vi "Wiimote Get Core Buttons, Acceleration, IR Sensor and Extension Controller.vi"(8 "error in":errorcluster, 11 "hWiimoteHandle in":u32 format="%08x") -> (0 "error out":errorcluster, 2 "Data out":T6, 3 "hWiimoteHandle out":u32 format="%08x")   [LabVIEW 2012, in "Wiimote.lvlib"]
uses:
  Wiimote.lvlib
  Wiimote Buttons.ctl
  Wiimote Acceleration.ctl
  Wiimote IR Sensor.ctl
  Wiimote Point.ctl
  Nunchuk Buttons.ctl
  Wiimote Reporting Mode.ctl
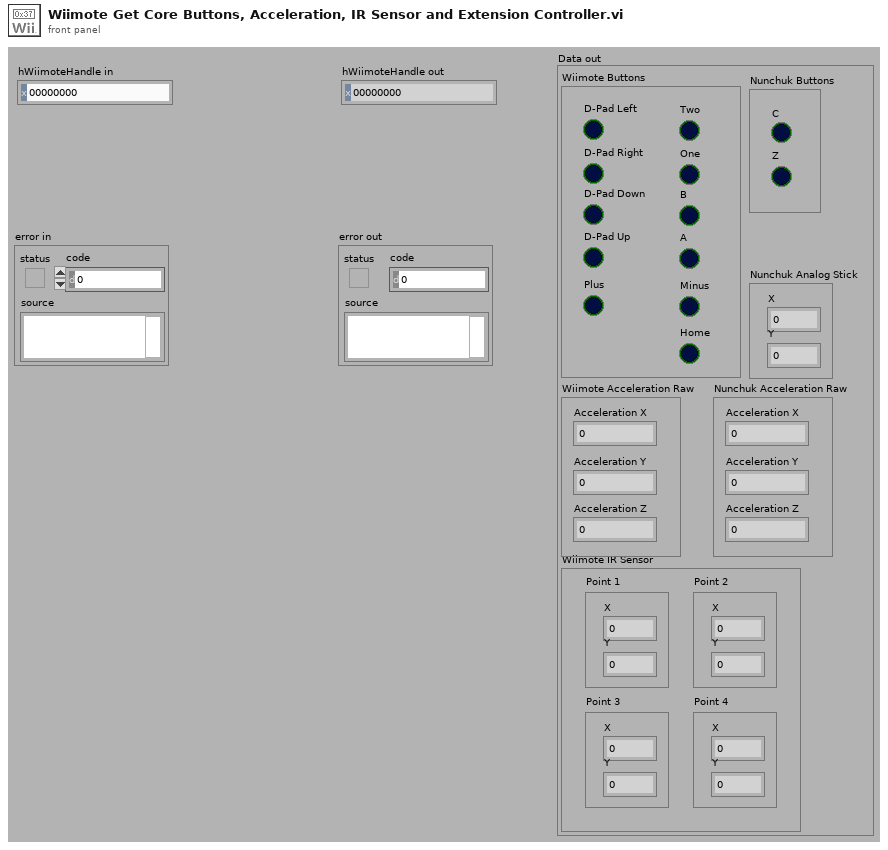
[diagram p1: front panel]
types:
  T1 = typedef "Wiimote.lvlib/Wiimote Buttons.ctl" = cluster{"D-Pad Left":bool, "D-Pad Right":bool, "D-Pad Down":bool, "D-Pad Up":bool, "Plus":bool, "Two":bool, "One":bool, "B":bool, "A":bool, "Minus":bool, "Home":bool}
  T2 = typedef "Wiimote.lvlib/Wiimote Acceleration.ctl" = cluster{"Acceleration X":dbl, "Acceleration Y":dbl, "Acceleration Z":dbl}
  T3 = typedef "Wiimote.lvlib/Wiimote IR Sensor.ctl" = cluster{"Point 1":T4, "Point 2":T4, "Point 3":T4, "Point 4":T4}
  T4 = typedef "Wiimote.lvlib/Wiimote Point.ctl" = cluster{"X":u16, "Y":u16}
  T5 = typedef "Wiimote.lvlib/Nunchuk Buttons.ctl" = cluster{"C":bool, "Z":bool}
  T6 = cluster{"Wiimote Buttons":T1, "Wiimote Acceleration Raw":T2, "Wiimote IR Sensor":T3, "Nunchuk Analog Stick":T4, "Nunchuk Acceleration Raw":T2, "Nunchuk Buttons":T5}
  T7 = typedef "Wiimote.lvlib/Wiimote Reporting Mode.ctl" = u8
  T8 = cluster{"Wiimote Buttons out":T1, "Wiimote Acceleration Raw out":T2, "Wiimote IR Sensor out":T3, "Nunchuk Analog Stick out":T4, "Nunchuk Acceleration Raw out":T2, "Nunchuk Buttons out":T5}
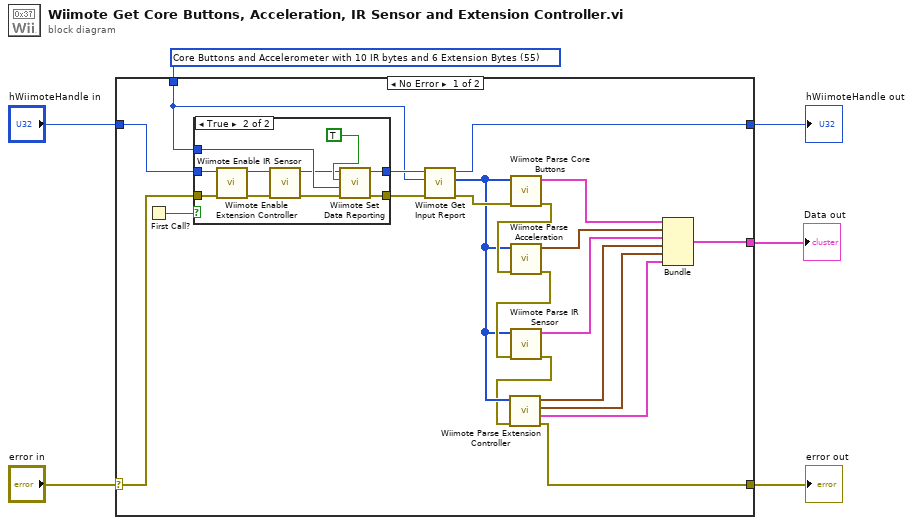
[diagram p0: block diagram]
diagram:
  w2 = T7 55 items=["Core Buttons"=48, "Core Buttons and Accelerometer"=49, "Core Buttons with 8 Extension bytes"=50, "Core Buttons and Accelerometer with 12 IR bytes"=51, "Core Buttons with 19 Extension bytes"=52, "Core Buttons and Accelerometer with 16 Extension Bytes"=53, "Core Buttons with 10 IR bytes and 9 Extension Bytes"=54, "Core Buttons and Accelerometer with 10 IR bytes and 6 Extension Bytes"=55] ("Reporting Mode")
  n1 = case shown="No Error" "error in" {
    selector: "error in" -> [w19 w40]
    tunnel: [w14 w40] -> w5
    tunnel: "hWiimoteHandle in" -> [w20 w39]
    tunnel: [w25 w39] -> w3
    tunnel: w2 -> [w21 _]
    tunnel: [w7 _] -> w1
    frame No Error {
      n2 = First Call?() -> (First Call?: T/F=w18:bool)
      n3 = case shown="True" w18 {
        tunnel: [w28 w33] -> w23
        tunnel: [w27 w29] -> w22
        tunnel: w21 -> [_ w38]
        tunnel: w20 -> [w28 w36]
        tunnel: w19 -> [w27 w32]
        frame False {
        }
        frame True {
          n4 = call "Wiimote Enable Extension Controller.vi"("error in"=w32, "hWiimoteHandle in"=w36) -> ("error out"=w31:errorcluster, "hWiimoteHandle out"=w35:u32)  [unwired: 8 in]
          n5 = call "Wiimote Enable IR Sensor.vi"("error in"=w31, "hWiimoteHandle in"=w35) -> ("error out"=w30:errorcluster, "hWiimoteHandle out"=w34:u32)  [unwired: 8 in]
          n6 = call "Wiimote Set Data Reporting.vi"("error in"=w30, "Reporting Mode"=w38, "Continuous"=TRUE, "hWiimoteHandle in"=w34) -> ("error out"=w29:errorcluster, "hWiimoteHandle out"=w33:u32)  [unwired: 6 in]
        }
      }
      n7 = call "Wiimote Get Input Report.vi"("error in"=w22, "bInputReport"=w21, "hWiimoteHandle in"=w23) -> ("error out"=w26:errorcluster, "pReportBuffer out"=w16:u8[], "hWiimoteHandle out"=w25:u32)  [unwired: 6 in]
      n8 = call "Wiimote Parse Core Buttons.vi"("error in"=w26, "pReportBuffer in"=w16) -> ("error out"=w24:errorcluster, "Wiimote Buttons out"=w13:T1)  [unwired: 8 in]
      n9 = call "Wiimote Parse Acceleration.vi"("error in"=w24, "pReportBuffer in"=w16) -> ("error out"=w17:errorcluster, "Wiimote Acceleration Raw out"=w12:T2)  [unwired: 8 in]
      n10 = call "Wiimote Parse IR Sensor.vi"("error in"=w17, "pReportBuffer in"=w16) -> ("error out"=w15:errorcluster, "Wiimote IR Sensor out"=w11:T3)  [unwired: 8 in]
      n11 = call "Wiimote Parse Extension Controller.vi"("error in"=w15, "pReportBuffer in"=w16) -> ("error out"=w14:errorcluster, "Nunchuk Buttons out"=w8:T5, "Nunchuk Acceleration Raw out"=w9:T2, "Nunchuk Analog Stick out"=w10:T4)  [unwired: 6 in]
      n12 = Bundle("Wiimote Buttons out"=w13, "Wiimote Acceleration Raw out"=w12, "Wiimote IR Sensor out"=w11, "Nunchuk Analog Stick out"=w10, "Nunchuk Acceleration Raw out"=w9, "Nunchuk Buttons out"=w8) -> (w7:T8)  [unwired: 1 in]
    }
    frame Error {
    }
  }
  "error out" <- w5
  "hWiimoteHandle out" <- w3
  "Data out" <- w1
